vi "Swerve Drive.vi"(0 "X":dbl(slide) scale=-1.0..1.0, 1 "Rot. Point Y":dbl, 3 "Rot. Point X":dbl, 7 "Y":dbl(slide) scale=1.0..-1.0, 11 "Z":dbl(knob) scale=1.0..-1.0, 12 "Auto Controls":bool, 13 "Robot-Centric":bool) -> ()   [LabVIEW 2013]
doc: "Main block for a swerve drive. X, Y, and Z are the only inputs that must be wired.\nX and Y are the joystick axes for translational (strafing) movement. Z is the joystick axis for rotation. Rotation point is the point relative to the center of the robot (in inches), around which the robot rotates. This input is optional, leave it blank to always rotate around the center of the robot. If Auto Controls is true, then the inputs will not be squared, and there will be no deadband. If Robot-Centric is true, then the gyro will be ignored, and pushing forward on the joystick will result in a foward movement relative to the robot's direction."
panel:
  in  "Robot Length":dbl=27.5
  in  "Robot Width":dbl=28.0
  # "SWERVE DRIVE\nVersion 3.1\n\nCory Lynch\nApple Pi Robotics\nTeam 2067"
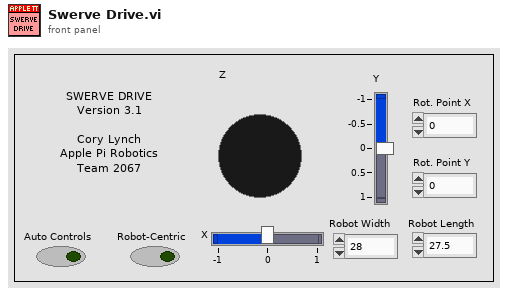
[diagram p1: front panel]
types:
  T1 = enum16{"Back Left", "Back Right", "Front Left", "Front Right"}
  T2 = typedef "WPI_MotorControlDeviceRef.ctl" = cluster{"DeviceStatus":errorcluster, "Type":enum16{"PWM", "CAN"}, "PWM":cluster{"Digital Module":T3, "PWM Channel":T4, "DeadBand":T5}, "CAN":cluster{"Device Number":u8, "Control Mode":T6, "Semaphore":T7, "Max Vout":dbl}, "Invert":bool, "TransformRef":T8, "InvTransformRef":T8}
  T3 = typedef "FPGA_TypedefDigitalModule.ctl" = enum16{"Digital Module 1", "Digital Module 2"}
  T4 = typedef "FPGA_DIOPWMChannel.ctl" = enum8{"PWM 1", "PWM 2", "PWM 3", "PWM 4", "PWM 5", "PWM 6", "PWM 7", "PWM 8", "PWM 9", "PWM 10", "Invalid"}
  T5 = typedef "WPI_PWMDeadband.ctl" = cluster{"Name":string, "maxPositivePwm":i32, "minPositivePwm":i32, "centerPwm":i32, "maxNegativePwm":i32, "minNegativePwm":i32, "angularRange":u16}
  T6 = typedef "WPI_CANJaguar_ControlMode.ctl" = enum8{"Percent VBus", "Current", "Speed", "Position", "Voltage"}
  T7 = typedef "Semaphore RefNum" = refnum<k1>
  T8 = typedef "WPI_PWMTransform_ConPane.ctl" = refnum<vi>
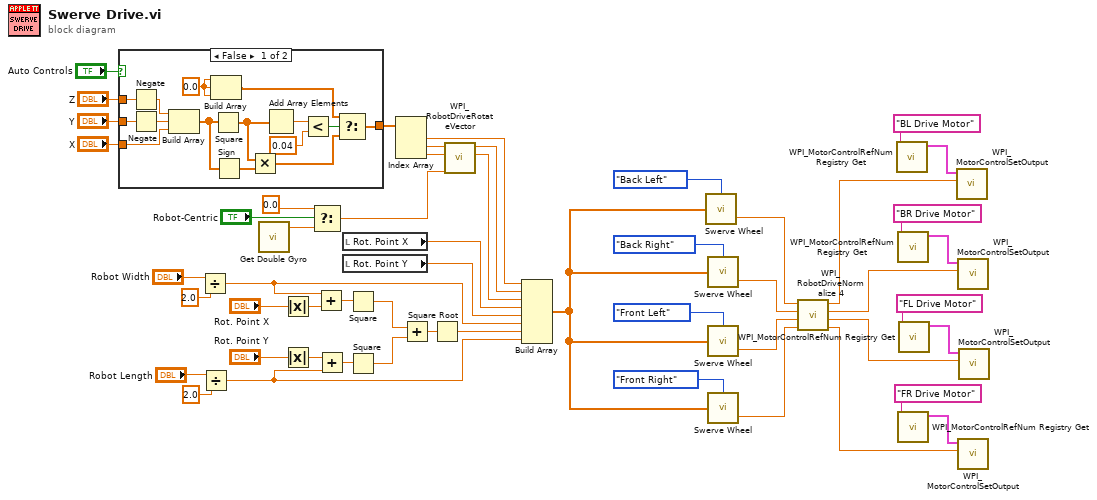
[diagram p0: block diagram]
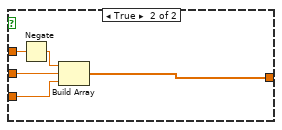
[diagram p2: hidden frame]
diagram:
  n1 = case shown="False" "Auto Controls" {
    tunnel: "Y" -> [w65 w70]
    tunnel: "X" -> [w59 w73]
    tunnel: "Z" -> [w58 w72]
    tunnel: [w55 w69] -> w10
    frame False {
      w63 = 0.0 ("element")
      n2 = Negate(x=w58) -> (-x=w54:dbl)
      n3 = Negate(x=w65) -> (-x=w57:dbl)
      n4 = Build Array(w54, w57, w59) -> (w62:dbl[])
      n5 = Build Array(w63, w63, w63) -> (w64:dbl[])
      n6 = Square(x=w62) -> (x^2=w60:dbl[])
      n7 = Sign(1:w62) -> (0:w61:dbl[])
      n8 = Multiply(x=w60, y=w61) -> (x*y=w56:dbl[])
      n9 = Add Array Elements(numeric array=w60) -> (sum=w68:dbl)
      n10 = Less?(x=w68, y=0.04 ("x")) -> (x < y?=w66:bool)
      n11 = Select(t=w64, s=w66, f=w56) -> (s? t:f=w55:dbl[])
    }
    frame True {
      n12 = Negate(x=w72) -> (-x=w71:dbl)
      n13 = Build Array(w71, w70, w73) -> (w69:dbl[])
    }
  }
  n14 = Divide(x="Robot Width", y=2.0) -> (x/y=w14:dbl)
  n15 = Divide(x="Robot Length", y=2.0) -> (x/y=w12:dbl)
  n16 = call "Get Double Gyro.vi"() -> ("Angle"=w6:dbl)  [unwired: 10 in, 1 out]
  n17 = Absolute Value(x="Rot. Point X") -> (abs(x)=w32:dbl)
  n18 = Absolute Value(x="Rot. Point Y") -> (abs(x)=w30:dbl)
  n19 = Select(t=0.0, s="Robot-Centric", f=w6) -> (s? t:f=w4:dbl)
  n20 = Add(x=w14, y=w32) -> (x+y=w31:dbl)
  n21 = Add(x=w30, y=w12) -> (x+y=w29:dbl)
  n22 = local read "Rot. Point X"() -> (w16:dbl)
  n23 = local read "Rot. Point Y"() -> (w15:dbl)
  n24 = Square(x=w31) -> (x^2=w27:dbl)
  n25 = Square(x=w29) -> (x^2=w28:dbl)
  n26 = Index Array(array=w10) -> (element #1=w3:dbl, element #2=w11:dbl, element #3=w19:dbl)  [unwired: 3 in]
  n27 = Add(x=w27, y=w28) -> (x+y=w26:dbl)
  n28 = Square Root(x=w26) -> (sqrt(x)=w13:dbl)
  n29 = call <vilib>:"WPI_RobotDriveRotateVector.vi"("Angle"=w4, "X"=w19, "Y"=w11) -> ("X'"=w8:dbl, "Y'"=w2:dbl)  [unwired: 7 out]
  n30 = Build Array(w3, w2, w8, w16, w15, w14, w13, w12) -> (w9:dbl[])
  n31 = call "Swerve Wheel.vi"("Wheel"=T1."Back Left", "Inputs"=w9) -> ("Speed"=w50:dbl)  [unwired: 3 in]
  n32 = call "Swerve Wheel.vi"("Wheel"=T1."Back Right", "Inputs"=w9) -> ("Speed"=w49:dbl)  [unwired: 3 in]
  n33 = call "Swerve Wheel.vi"("Wheel"=T1."Front Left", "Inputs"=w9) -> ("Speed"=w48:dbl)  [unwired: 3 in]
  n34 = call "Swerve Wheel.vi"("Wheel"=T1."Front Right", "Inputs"=w9) -> ("Speed"=w47:dbl)  [unwired: 3 in]
  n35 = call <vilib>:"WPI_RobotDriveNormalize 4.vi"("D"=w47, "C"=w48, "B"=w49, "A"=w50) -> ("D'"=w34:dbl, "C'"=w35:dbl, "B'"=w36:dbl, "A'"=w37:dbl)
  n36 = call <vilib>:"WPI_MotorControlRefNum Registry Get.vi"("refnum name"="BL Drive Motor") -> ("MotorControlDevRef"=w45:T2)  [unwired: 9 in, 1 out]
  n37 = call <vilib>:"WPI_MotorControlRefNum Registry Get.vi"("refnum name"="BR Drive Motor") -> ("MotorControlDevRef"=w42:T2)  [unwired: 9 in, 1 out]
  n38 = call <vilib>:"WPI_MotorControlRefNum Registry Get.vi"("refnum name"="FR Drive Motor") -> ("MotorControlDevRef"=w38:T2)  [unwired: 9 in, 1 out]
  n39 = call <vilib>:"WPI_MotorControlRefNum Registry Get.vi"("refnum name"="FL Drive Motor") -> ("MotorControlDevRef"=w41:T2)  [unwired: 9 in, 1 out]
  n40 = call <vilib>:"WPI_MotorControlSetOutput.vi"("Output"=w37, "MotorControlDevRef"=w45) -> ()  [unwired: 7 in, 3 out]
  n41 = call <vilib>:"WPI_MotorControlSetOutput.vi"("Output"=w36, "MotorControlDevRef"=w42) -> ()  [unwired: 7 in, 3 out]
  n42 = call <vilib>:"WPI_MotorControlSetOutput.vi"("Output"=w34, "MotorControlDevRef"=w38) -> ()  [unwired: 7 in, 3 out]
  n43 = call <vilib>:"WPI_MotorControlSetOutput.vi"("Output"=w35, "MotorControlDevRef"=w41) -> ()  [unwired: 7 in, 3 out]
